vi "test Add and Remove GE Reflective Memory.vi"(8 "error in (no error)":errorcluster, 11 "TestCase in":refnum<class "Add and Remove Test.lvclass">) -> (0 "error out":errorcluster, 3 "TestCase out":refnum<class "Add and Remove Test.lvclass">)   [LabVIEW 2020, in "Add and Remove Test.lvclass"]
uses:
  Add and Remove Test.lvclass
  Includes/DSF Core.lvlibp/Typedefs/DSF Engine Framework Configuration.ctl
  Includes/DSF Core.lvlibp/Typedefs/DSF Engine Plugin Configuration.ctl
  Includes/DSF Core.lvlibp/Typedefs/Core Plugin Configuration.ctl
  Includes/DSF Core.lvlibp/Typedefs/DSF Timing Info.ctl
  Includes/DSF Core.lvlibp/Typedefs/DSF Settings Info.ctl
  Includes/DSF Core.lvlibp/Typedefs/DSF Engine Plugin Thread Configuration.ctl
  Includes/DSF Core.lvlibp/Typedefs/Core Thread Configuration.ctl
  Includes/DSF Core.lvlibp/Typedefs/DSF Engine Transfer Group Configuration.ctl
  Includes/DSF Core.lvlibp/Typedefs/Core Group Configuration.ctl
  Includes/DSF Core.lvlibp/Typedefs/DSF Direction.ctl
  Includes/DSF Core.lvlibp/Typedefs/DSF Timeout Behavior.ctl
  Includes/DSF Core.lvlibp/Typedefs/DSF Engine Transfer Configuration.ctl
  Includes/DSF Core.lvlibp/Typedefs/Core Transfer Configuration.ctl
  Includes/DSF Core.lvlibp/Typedefs/DSF Engine Channel Configuration.ctl
  Includes/DSF Core.lvlibp/Typedefs/Core Channel Configuration.ctl
  Includes/DSF Core.lvlibp/Typedefs/DSF Data Type.ctl
  <vilib>/NI VeriStand/Custom Device API/Custom Device Item Ref.ctl
  Add and Remove Test.lvclass/Add and Remove Test.ctl
  <vilib>/addons/_JKI Toolkits/VI Tester/TestCase.llb/TestCase.lvclass
  Scripting API/Data Sharing Framework Custom Device Scripting.lvlib
  Includes/DSF Core.lvlibp
  Includes/DSF Core.lvlibp/Classes/Configuration/Core/Plugin/Plugin Configuration.lvclass
  Includes/DSF Core.lvlibp/Classes/Configuration/Core/Thread/Thread Configuration.lvclass
  Includes/DSF Core.lvlibp/Classes/Configuration/Core/Group/Group Configuration.lvclass
  Includes/DSF Core.lvlibp/Classes/Configuration/Core/Transfer/Transfer Configuration.lvclass
  Includes/DSF Core.lvlibp/Classes/Configuration/Core/Channel/Channel Configuration.lvclass
  <vilib>/NI/VeriStand Custom Device Testing Tools/VeriStandTestUtilities/VeriStandTestUtilities.lvlib
  Includes/DSF Core.lvlibp/Classes/Configuration Session/Configuration Session.lvclass
  <vilib>/NI VeriStand/Custom Device API/Custom Device API.lvlib
  C:/Program Files (x86)/National Instruments/LabVIEW 2020/vi.lib/addons/_JKI Toolkits/VI Tester/TestCase.llb/TestCase.lvclass
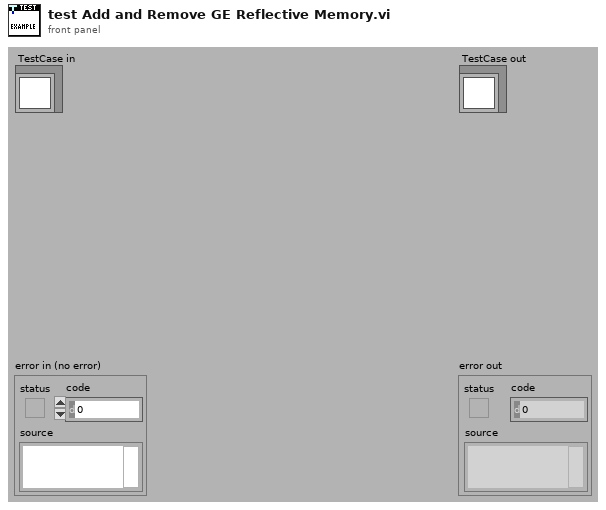
[diagram p1: front panel]
types:
  T1 = typedef "DSF Core.lvlibp/DSF Engine Framework Configuration.ctl" = cluster{"plugins":T2[]}
  T2 = typedef "DSF Core.lvlibp/DSF Engine Plugin Configuration.ctl" = cluster{"core":T3, "component settings":T5[], "threads":T6[]}
  T3 = typedef "DSF Core.lvlibp/Plugin Configuration.lvclass/Core Plugin Configuration.ctl" = cluster{"name":string, "components":string[], "cycle timing":T4}
  T4 = typedef "DSF Core.lvlibp/DSF Timing Info.ctl" = cluster{"priority":u64, "decimation":u64, "offset":u64}
  T5 = typedef "DSF Core.lvlibp/DSF Settings Info.ctl" = cluster{"component":string, "values":cluster{"key":string, "value":string}[]}
  T6 = typedef "DSF Core.lvlibp/DSF Engine Plugin Thread Configuration.ctl" = cluster{"core":T7, "component settings":T5[], "transfer groups":T8[]}
  T7 = typedef "DSF Core.lvlibp/Thread Configuration.lvclass/Core Thread Configuration.ctl" = cluster{"processor":i32, "priority offset":i16}
  T8 = typedef "DSF Core.lvlibp/DSF Engine Transfer Group Configuration.ctl" = cluster{"core":T9, "component settings":T5[], "transfers":T12[]}
  T9 = typedef "DSF Core.lvlibp/Group Configuration.lvclass/Core Group Configuration.ctl" = cluster{"name":string, "direction":T10, "cycle timing":T4, "timeout behavior":T11, "enable conversion":bool}
  T10 = typedef "DSF Core.lvlibp/DSF Direction.ctl" = enum8{"Tx", "Rx"}
  T11 = typedef "DSF Core.lvlibp/DSF Timeout Behavior.ctl" = enum8{"Increment Late Count", "Throw Error"}
  T12 = typedef "DSF Core.lvlibp/DSF Engine Transfer Configuration.ctl" = cluster{"core":T13, "component settings":T5[], "channels":T14[]}
  T13 = typedef "DSF Core.lvlibp/Transfer Configuration.lvclass/Core Transfer Configuration.ctl" = cluster{"name":string}
  T14 = typedef "DSF Core.lvlibp/DSF Engine Channel Configuration.ctl" = cluster{"core":T15, "component settings":T5[]}
  T15 = typedef "DSF Core.lvlibp/Channel Configuration.lvclass/Core Channel Configuration.ctl" = cluster{"name":string, "units":string, "engine data type":T16, "string data type":T16, "string offset":u64}
  T16 = typedef "DSF Core.lvlibp/DSF Data Type.ctl" = enum8{"Bool", "SGL", "DBL", "I8", "I16", "I32", "I64", "U8", "U16", "U32", "U64"}
  T17 = typedef "Custom Device API.lvlib/Custom Device Item Ref.ctl" = u64
  T18 = typedef "DSF Core.lvlibp/DSF Version Info.ctl" = cluster{"major":u32, "minor":u32, "fix":u32, "build":string}
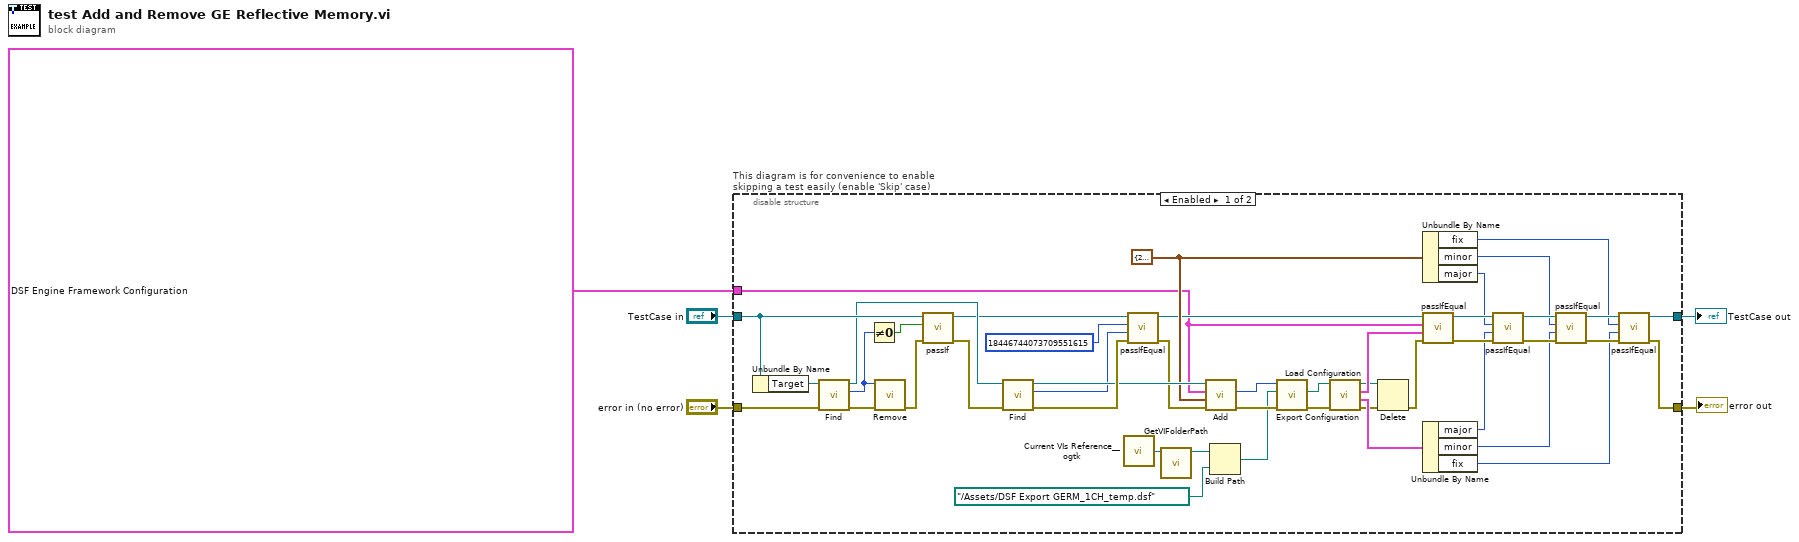
[diagram p0: block diagram]
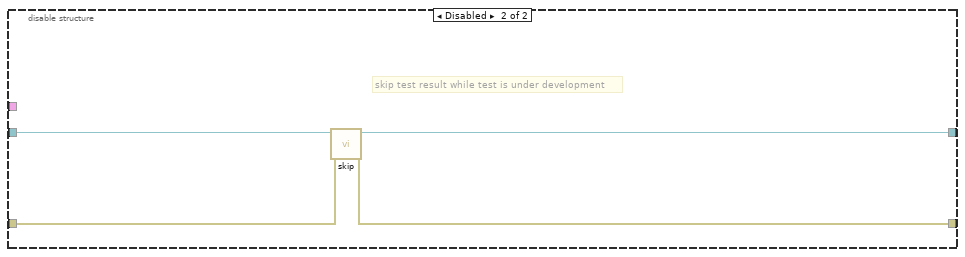
[diagram p2: hidden frame]
diagram:
  n1 = disable-structure "This diagram is for convenience to enable skipping a test easily (enable 'Skip' case)" shown="Enabled" {
    disable-tunnel: "TestCase in" -> [w50 w54]
    disable-tunnel: [w20 w52] -> w2
    disable-tunnel: [w11 w53] -> w4
    disable-tunnel: "error in (no error)" -> [w48 w51]
    disable-tunnel: T1 {"plugins"=[{"core"={"name"="", "components"=["GE Reflective Memory"], "cycle timing"={"priority"=10000, "decimation"=1, "offset"=0}}, "component settings"=[], "threads"=[{"core"={"processor"=-2, "priority offset"=0}, "component settings"=[], "transfer groups"=[{"core"={"name"="Group", "direction"=enum."Tx", "cycle timing"={"priority"=100, "decimation"=1, "offset"=0}, "timeout behavior"=enum."Increment Late Count", "enable conversion"=FALSE}, "component settings"=[], "transfers"=[{"core"={"name"="Transfer"}, "component settings"=[], "channels"=[{"core"={"name"="Voltage", "units"="V", "engine data type"=enum."DBL", "string data type"=enum."DBL", "string offset"=0}, "component settings"=[]}]}]}, {"core"={"name"="Group", "direction"=enum."Rx", "cycle timing"={"priority"=100, "decimation"=1, "offset"=0}, "timeout behavior"=enum."Increment Late Count", "enable conversion"=FALSE}, "component settings"=[], "transfers"=[{"core"={"name"="Transfer"}, "component settings"=[], "channels"=[{"core"={"name"="Voltage", "units"="V", "engine data type"=enum."DBL", "string data type"=enum."DBL", "string offset"=0}, "component settings"=[]}]}]}]}]}]} ("framework configuration") -> [w18 _]
    frame Enabled {
      w28 = cluster{"major":u32, "minor":u32, "fix":u32} {"major"=2020, "minor"=3, "fix"=33} ("configuration version")
      n2 = Unbundle By Name(w50) -> ("Target"=w49:refnum<k24>)
      n3 = call "Find.vi"("error in"=w48, "target in"=w49) -> ("error out"=w45:errorcluster, "data sharing framework custom device"=w46:T17, "target out"=w44:refnum<k24>)  [unwired: 6 in, 1 out]
      n4 = Not Equal To 0?(x=w46) -> (x != 0?=w47:bool)
      n5 = call "Remove.vi"("error in"=w45, "data sharing framework custom device"=w46) -> ("error out"=w43:errorcluster)  [unwired: 9 in]
      n6 = call-dynamic "passIf.vi"("error in (no error)"=w43, "pass"=w47, "TestCase in"=w50) -> ("error out"=w42:errorcluster, "TestCase out"=w41:refnum<class "Add and Remove Test.lvclass">)  [unwired: 7 in]
      n7 = call "Find.vi"("error in"=w42, "target in"=w44) -> ("error out"=w40:errorcluster, "data sharing framework custom device"=w7:T17, "target out"=w39:refnum<k24>)  [unwired: 6 in, 1 out]
      n8 = call <userlib>:"Current VIs Reference__ogtk.vi"() -> ("Current VI's reference"=w35:refnum<vi>)  [unwired: 5 in]
      n9 = call-dynamic "passIfEqual.vi"("error in (no error)"=w40, "y"=w7, "x"=T17 18446744073709551615 ("data sharing framework custom device"), "TestCase in"=w41) -> ("error out"=w38:errorcluster, "TestCase out"=w21:refnum<class "Add and Remove Test.lvclass">)  [unwired: 6 in]
      n10 = call <vilib>:"GetVIFolderPath.vi"("VI Reference in"=w35) -> ("VI Folder Path out"=w34:path)  [unwired: 9 in, 1 out]
      n11 = call "Add.vi"("error in"=w38, "configuration version"=w28, "framework configuration"=w18, "target in"=w39) -> ("error out"=w37:errorcluster, "data sharing framework custom device"=w36:T17)  [unwired: 5 in, 1 out]
      n12 = Build Path(base path=w34, name or relative path=path "../Assets/DSF Export GERM_1CH_temp.dsf" ("base path")) -> (appended path=w32:path)
      n13 = call "Export Configuration.vi"("error in"=w37, "configuration file path"=w32, "data sharing framework custom device"=w36) -> ("error out"=w30:errorcluster, "actual configuration file path"=w31:path)  [unwired: 6 in, 1 out]
      n14 = call "Load Configuration.vi"("error in (no error)"=w30, "configuration file path"=w31) -> ("error out"=w10:errorcluster, "version"=w29:T18, "framework configuration"=w19:T1, "configuration file path dup"=w8:path)  [unwired: 6 in]
      n15 = Delete(path (use dialog)=w8, error in=w10) -> (error out=w9:errorcluster)  [unwired: 3 in, 2 out]
      n16 = Unbundle By Name(w28) -> ("fix"=w14:u32, "minor"=w12:u32, "major"=w13:u32)
      n17 = call-dynamic "passIfEqual.vi"("error in (no error)"=w9, "y"=w19, "x"=w18, "TestCase in"=w21) -> ("error out"=w26:errorcluster, "TestCase out"=w27:refnum<class "Add and Remove Test.lvclass">)  [unwired: 6 in]
      n18 = Unbundle By Name(w29) -> ("major"=w17:u32, "minor"=w16:u32, "fix"=w15:u32)
      n19 = call-dynamic "passIfEqual.vi"("error in (no error)"=w26, "y"=w17, "x"=w13, "TestCase in"=w27) -> ("error out"=w24:errorcluster, "TestCase out"=w25:refnum<class "Add and Remove Test.lvclass">)  [unwired: 6 in]
      n20 = call-dynamic "passIfEqual.vi"("error in (no error)"=w24, "y"=w16, "x"=w12, "TestCase in"=w25) -> ("error out"=w22:errorcluster, "TestCase out"=w23:refnum<class "Add and Remove Test.lvclass">)  [unwired: 6 in]
      n21 = call-dynamic "passIfEqual.vi"("error in (no error)"=w22, "y"=w15, "x"=w14, "TestCase in"=w23) -> ("error out"=w11:errorcluster, "TestCase out"=w20:refnum<class "Add and Remove Test.lvclass">)  [unwired: 6 in]
    }
    frame Disabled {
      # "skip test result while test is under development"
      n22 = call <vilib>:"skip.vi"("error in (no error)"=w51, "TestCase in"=w54) -> ("error out"=w53:errorcluster, "TestCase out"=w52:refnum<class "Add and Remove Test.lvclass">)  [unwired: 8 in]
    }
  }
  "error out" <- w4
  "TestCase out" <- w2
